vi "Centauro_Button_Press.vi"(0 "GEA2 Reference In":refnum<k24>, 5 "GEA Inputs":T1={"Source"=228, "Destination"=37} {"Destination" format="%.0x"; "Source" format="%.0x"}, 7 "Board Index":i32, 9 "Button":T2, 11 "Error In":errorcluster, 12 "Hold Time (s)":dbl=0.5 format="%#_13g") -> (4 "GEA2 Reference Out":refnum<k24>, 15 "Error Out":errorcluster)   [LabVIEW 2016]
uses:
  Q:/Common/DLLs/GEA3/GeaCommunication.dll
  Common/DLLs/GEA3/GeaCommunication.dll
  Type Defs/JL_Buttons.ctl
  Common/LabVIEW GEA2 Toolkit/LabVIEW_GEA2_Toolkit.lvlibp/type defs/Source_Destination.ctl
  Common/LabVIEW GEA2 Toolkit/LabVIEW_GEA2_Toolkit.lvlibp/type defs/ERD Write Data In.ctl
  Common/LabVIEW GEA2 Toolkit/LabVIEW_GEA2_Toolkit.lvlibp/type defs/Data Type.ctl
  <vilib>/DAQmx/write.llb/DAQmx Write (Digital Bool 1Line 1Point).vi
  <vilib>/DAQmx/create/channels.llb/DAQmx Create Channel (DO-Digital Output).vi
  <vilib>/DAQmx/miscellaneous.llb/DAQmx Fill In Error Info.vi
  Common/LabVIEW GEA2 Toolkit/LabVIEW_GEA2_Toolkit.lvlibp
panel:
  in  "SLB?":bool=TRUE
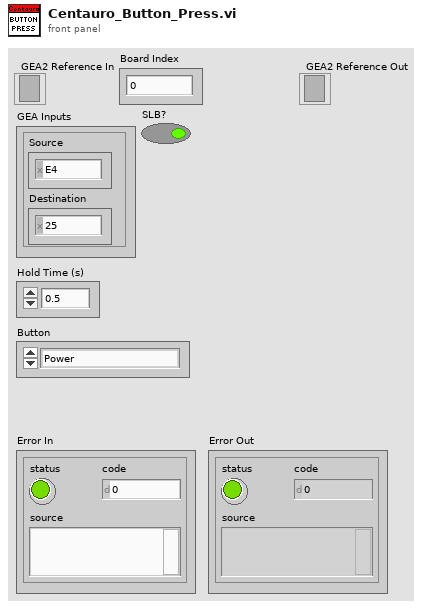
[diagram p1: front panel]
types:
  T1 = typedef "LabVIEW_GEA2_Toolkit.lvlibp/Source_Destination.ctl" = cluster{"Source":u8, "Destination":u8}
  T2 = typedef "JL_Buttons.ctl" = enum16{"Power", "Start / Pause ", "Temp Option ", "Dryness Level", "Time Option", "Time Increment ", "Time Decrement ", "MyCycle", "eDry ", "Delay", "Extended Tumble", "Control Lock", "Volume/Signal", "Damp Alert / Drum Light", "Unused", "(SW213)", "(SW322)", "Clear / Reset"}
  T3 = typedef "LabVIEW_GEA2_Toolkit.lvlibp/ERD Write Data In.ctl" = cluster{"ERD Number":u16, "Data Type":T4, "Data":string}
  T4 = typedef "LabVIEW_GEA2_Toolkit.lvlibp/Data Type.ctl" = enum16{"string", "boolean", "uint8_t", "uint16_t", "uint32_t", "uint64_t", "int8_t", "int16_t", "int32_t", "int64_t"}
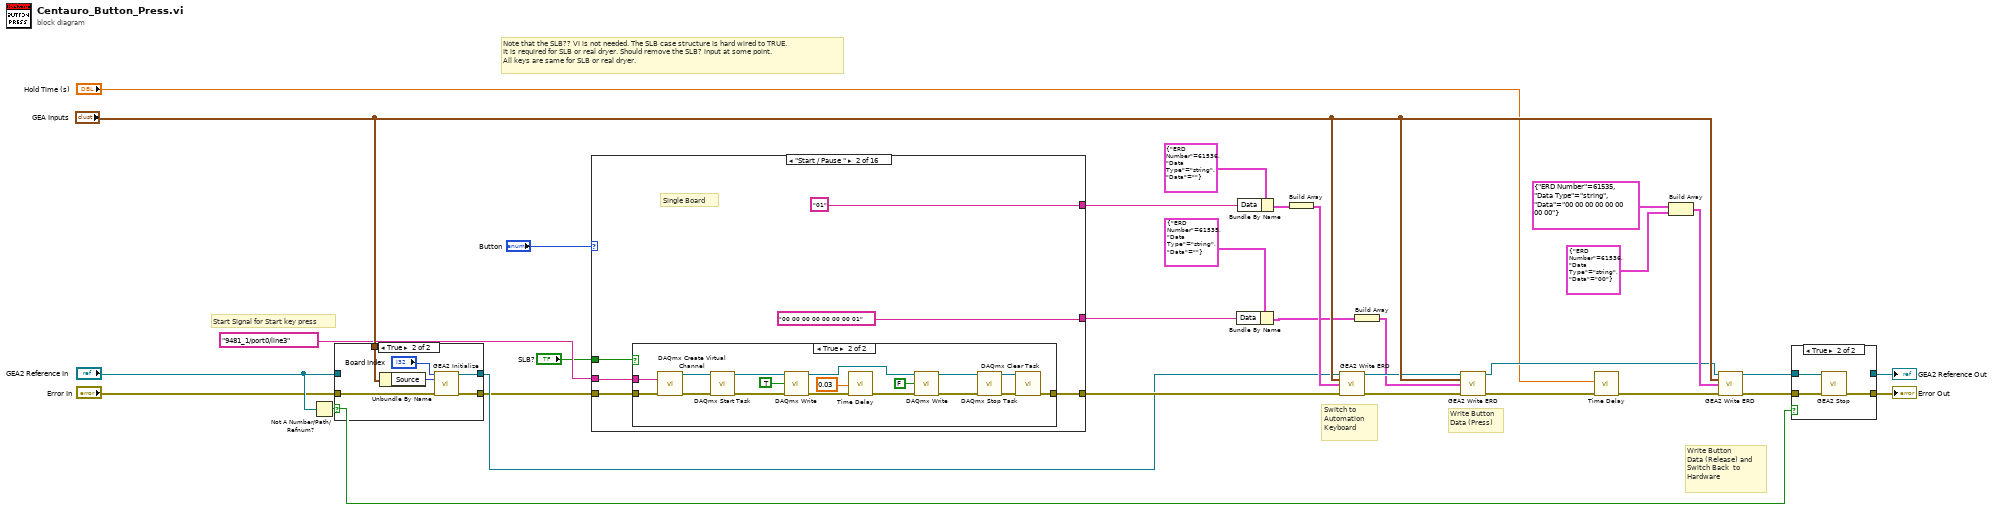
[diagram p0: block diagram]
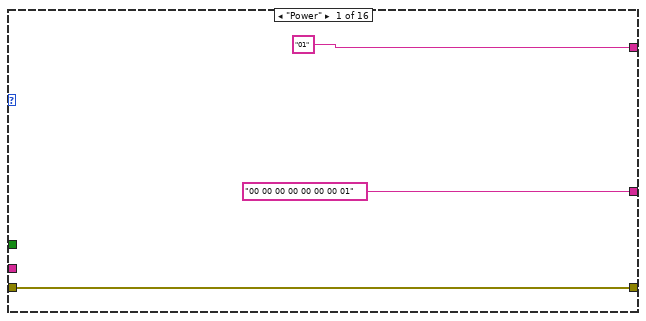
[diagram p2: hidden frame]
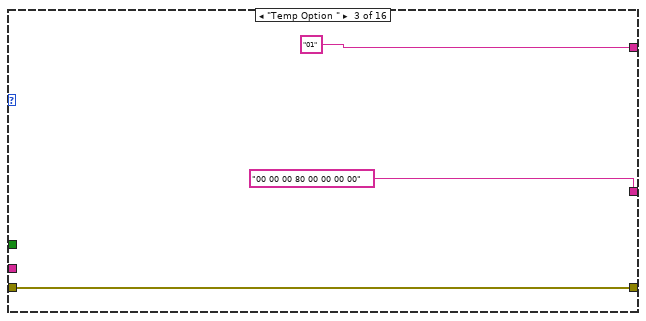
[diagram p4: hidden frame]
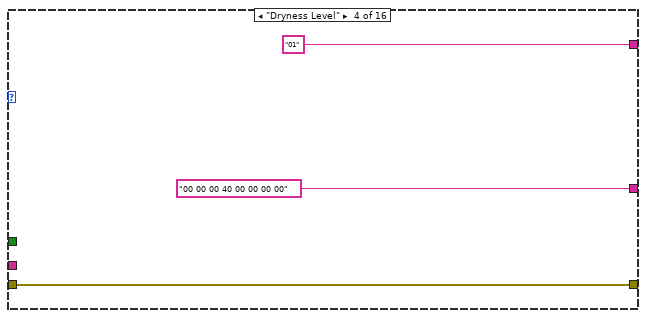
[diagram p5: hidden frame]
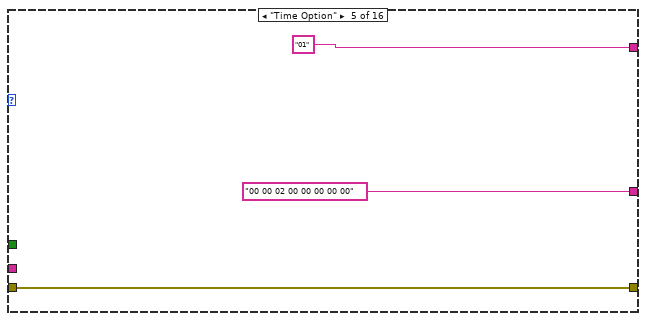
[diagram p6: hidden frame]
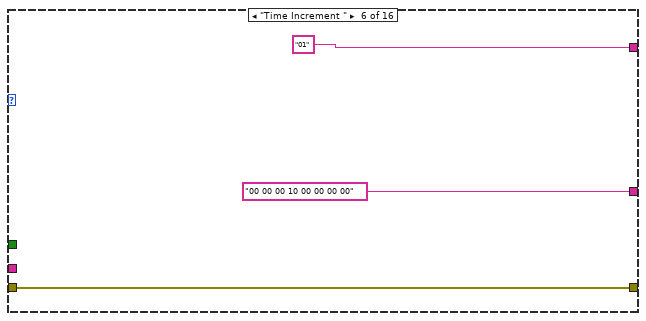
[diagram p7: hidden frame]
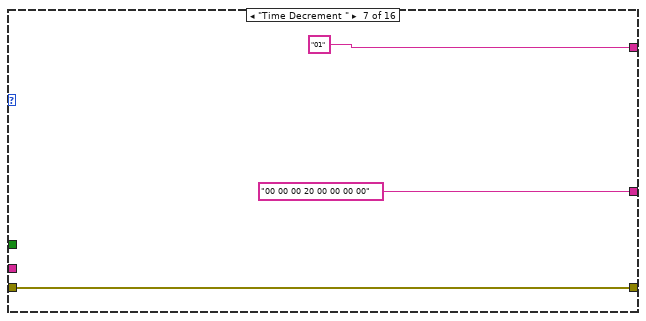
[diagram p8: hidden frame]
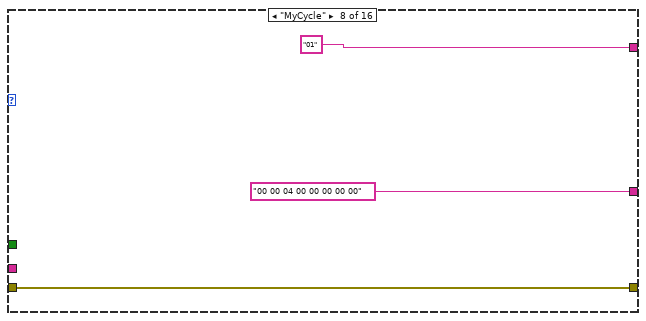
[diagram p9: hidden frame]
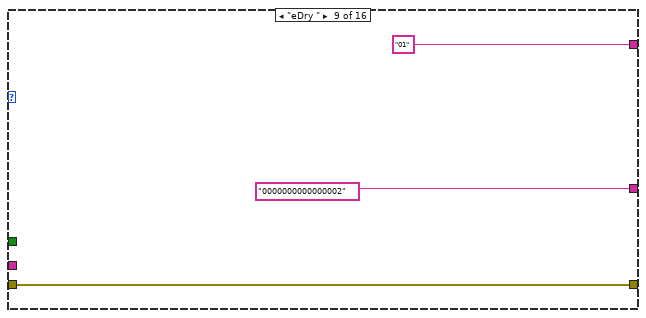
[diagram p10: hidden frame]
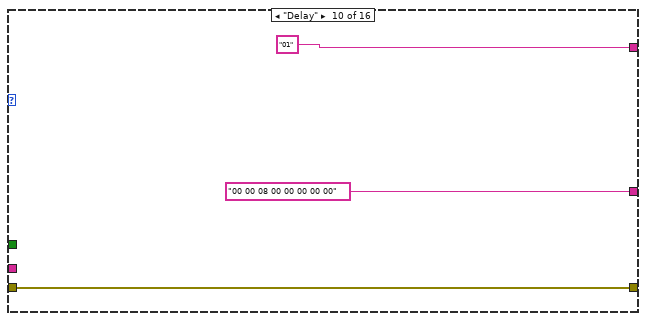
[diagram p11: hidden frame]
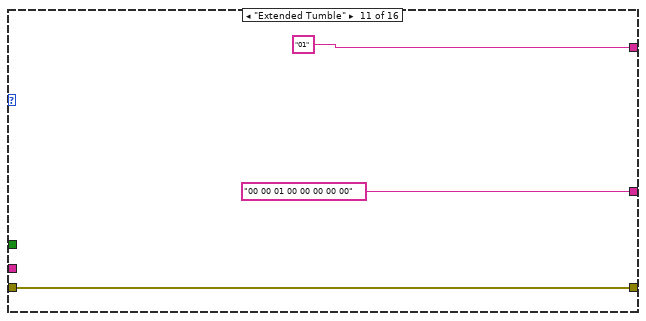
[diagram p12: hidden frame]
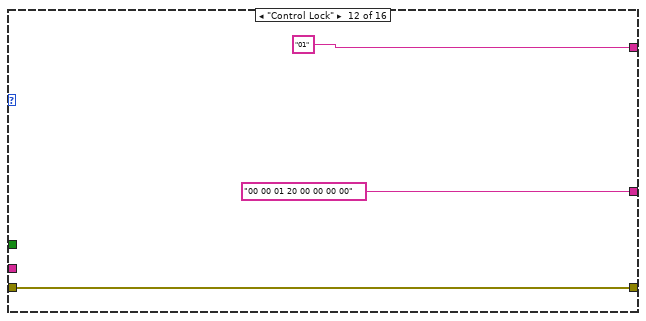
[diagram p13: hidden frame]
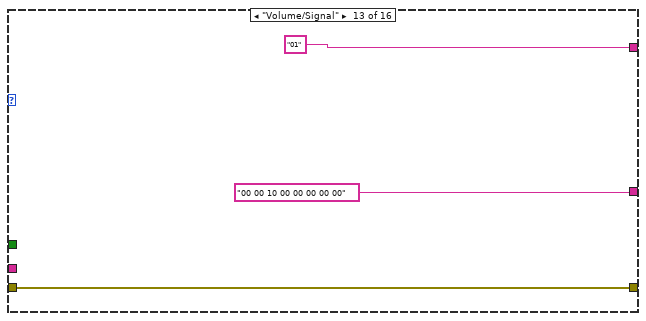
[diagram p14: hidden frame]
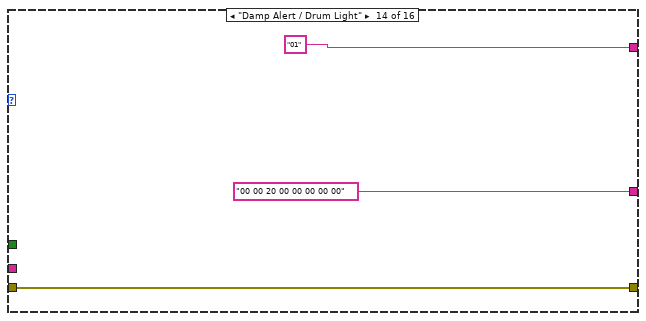
[diagram p15: hidden frame]
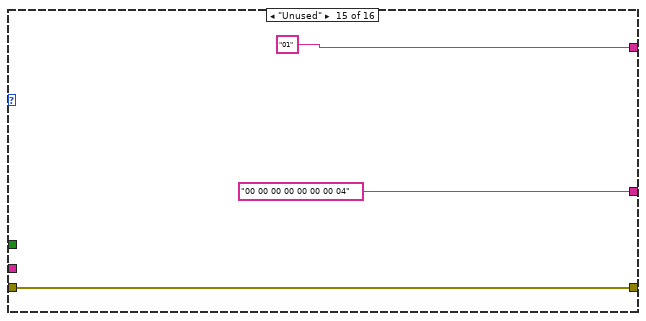
[diagram p16: hidden frame]
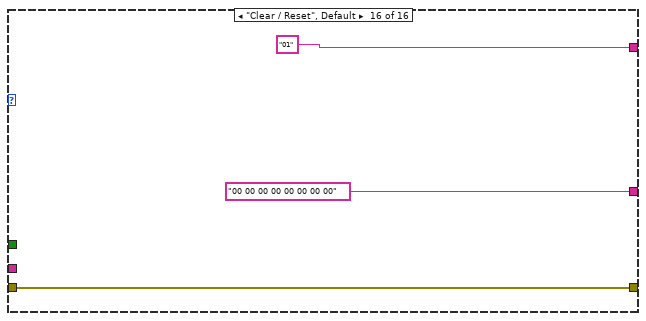
[diagram p17: hidden frame]
diagram:
  # "Note that the SLB?? VI is not needed. The SLB case structure is hard wired to TRUE.\nIt is required for SLB or real dryer. Should remove the SLB? input at some point.\nAll keys are same for SLB or real dryer."
  # "Start Signal for Start key press"
  # "Write Button\nData (Release) and \nSwitch Back  to\nHardware"
  # "Write Button\nData (Press)"
  # "Switch to\nAutomation \nKeyboard"
  n1 = Not A Number/Path/Refnum?(number/path/refnum="GEA2 Reference In") -> (NaN/Path/Refnum?=w28:bool)
  n2 = case shown="True" w28 {
    tunnel: "Error In" -> [w32 w39]
    tunnel: [w32 w38] -> w2
    tunnel: "GEA2 Reference In" -> [w33 _]
    tunnel: [w33 w37] -> w3
    tunnel: "GEA Inputs" -> [_ w35]
    frame False {
    }
    frame True {
      n3 = Unbundle By Name(w35) -> ("Source"=w36:u8)
      n4 = call "GEA2 Initialize.vi"("Board Index"="Board Index", "Source Address"=w36, "error in"=w39) -> ("GEA2 Reference Out"=w37:refnum<k24>, "error out"=w38:errorcluster)  [unwired: 10 in, 1 out]
    }
  }
  n5 = case shown="\"Start / Pause \"" "Button" {
    tunnel: ["01" "01" "01" "01" "01" "01" "01" "01" "01" "01" "01" "01" "01" "01" "01" "01"] -> w10
    tunnel: ["00 00 00 00 00 00 00 01" "00 00 00 00 00 00 00 01" "00 00 00 80 00 00 00 00" "00 00 00 40 00 00 00 00" "00 00 02 00 00 00 00 00" "00 00 00 10 00 00 00 00" "00 00 00 20 00 00 00 00" "00 00 04 00 00 00 00 00" "0000000000000002" "00 00 08 00 00 00 00 00" "00 00 01 00 00 00 00 00" "00 00 01 20 00 00 00 00" "00 00 10 00 00 00 00 00" "00 00 20 00 00 00 00 00" "00 00 00 00 00 00 00 04" "00 00 00 00 00 00 00 00"] -> w9
    tunnel: tag "9481_1/port0/line3" ("Line(s)") -> [_ w46 _ _ _ _ _ _ _ _ _ _ _ _ _ _]
    tunnel: [w40 w45 w67 w70 w73 w76 w79 w82 w85 w88 w91 w94 w97 w100 w103 w106] -> w4
    tunnel: w2 -> [w40 w44 w67 w70 w73 w76 w79 w82 w85 w88 w91 w94 w97 w100 w103 w106]
    tunnel: "SLB?" -> [_ w43 _ _ _ _ _ _ _ _ _ _ _ _ _ _]
    frame "Power" {
    }
    frame "Start / Pause " {
      # "Single Board"
      n6 = case shown="True" w43 {
        tunnel: w46 -> [_ w60]
        tunnel: [w49 w57] -> w45
        tunnel: w44 -> [w49 w53]
        frame False {
        }
        frame True {
          n7 = call-poly <vilib>:"DAQmx Create Virtual Channel.vi"("lines"=w60, "error in"=w53) -> ("task out"=w63:refnum<k21>, "error out"=w64:errorcluster)  [unwired: 12 in]
          n8 = call <vilib>:"DAQmx Start Task.vi"("task/channels in"=w63, "error in"=w64) -> ("task out"=w66:refnum<k21>, "error out"=w65:errorcluster)  [unwired: 12 in]
          n9 = call-poly <vilib>:"DAQmx Write.vi"("task/channels in"=w66, "data"=TRUE ("Boolean"), "error in"=w65) -> ("task out"=w54:refnum<k21>, "error out"=w56:errorcluster)  [unwired: 10 in, 1 out]
          n10 = call "Time Delay"("error in (no error)"=w56, "Delay Time (s)"=0.03) -> ("error out"=w55:errorcluster)  [unwired: 9 in]
          n11 = call-poly <vilib>:"DAQmx Write.vi"("task/channels in"=w54, "data"=FALSE ("Boolean"), "error in"=w55) -> ("task out"=w59:refnum<k21>, "error out"=w58:errorcluster)  [unwired: 10 in, 1 out]
          n12 = call <vilib>:"DAQmx Stop Task.vi"("task/channels in"=w59, "error in"=w58) -> ("task out"=w62:refnum<k21>, "error out"=w61:errorcluster)  [unwired: 12 in]
          n13 = call <vilib>:"DAQmx Clear Task.vi"("task in"=w62, "error in"=w61) -> ("error out"=w57:errorcluster)  [unwired: 13 in]
        }
      }
    }
    frame "Temp Option " {
    }
    frame "Dryness Level" {
    }
    frame "Time Option" {
    }
    frame "Time Increment " {
    }
    frame "Time Decrement " {
    }
    frame "MyCycle" {
    }
    frame "eDry " {
    }
    frame "Delay" {
    }
    frame "Extended Tumble" {
    }
    frame "Control Lock" {
    }
    frame "Volume/Signal" {
    }
    frame "Damp Alert / Drum Light" {
    }
    frame "Unused" {
    }
    frame "Clear / Reset", Default {
    }
  }
  n14 = Bundle By Name(cluster=T3 {"ERD Number"=61535, "Data Type"=enum."string", "Data"=""} ("ERD Write Data In"), "Data"=w9) -> (w14:T3)
  n15 = Bundle By Name(cluster=T3 {"ERD Number"=61536, "Data Type"=enum."string", "Data"=""} ("ERD Write Data In"), "Data"=w10) -> (w25:T3)
  n16 = Build Array(w25) -> (w24:T3[])
  n17 = call "GEA2 Write ERD.vi"("GEA2 Reference In"=w3, "GEA Inputs"="GEA Inputs", "Write ERD List"=w24, "Error In"=w4) -> ("GEA2 Reference Out"=w16:refnum<k24>, "Error Out"=w19:errorcluster)  [unwired: 9 in, 1 out]
  n18 = Build Array(w14) -> (w13:T3[])
  n19 = call "GEA2 Write ERD.vi"("GEA2 Reference In"=w16, "GEA Inputs"="GEA Inputs", "Write ERD List"=w13, "Error In"=w19) -> ("GEA2 Reference Out"=w15:refnum<k24>, "Error Out"=w18:errorcluster)  [unwired: 9 in, 1 out]
  n20 = call "Time Delay"("error in (no error)"=w18, "Delay Time (s)"="Hold Time (s)") -> ("error out"=w22:errorcluster)  [unwired: 9 in]
  n21 = Build Array(T3 {"ERD Number"=61535, "Data Type"=enum."string", "Data"="00 00 00 00 00 00 00 00"} ("ERD Write Data In"), T3 {"ERD Number"=61536, "Data Type"=enum."string", "Data"="00"} ("ERD Write Data In")) -> (w23:T3[])
  n22 = call "GEA2 Write ERD.vi"("GEA2 Reference In"=w15, "GEA Inputs"="GEA Inputs", "Write ERD List"=w23, "Error In"=w22) -> ("GEA2 Reference Out"=w20:refnum<k24>, "Error Out"=w21:errorcluster)  [unwired: 9 in, 1 out]
  n23 = case shown="True" w28 {
    tunnel: [w109 w113] -> w31
    tunnel: w20 -> [w110 w112]
    tunnel: [w110 _] -> w30
    tunnel: w21 -> [w109 w111]
    frame False {
    }
    frame True {
      n24 = call "GEA2 Stop.vi"("GEA2 Reference In"=w112, "Error In"=w111) -> ("Error Out"=w113:errorcluster)  [unwired: 13 in]
    }
  }
  "Error Out" <- w31
  "GEA2 Reference Out" <- w30
